vi "G4BaseTemplate_Singleton_4x4x4_GetInstance.vi"(8 "error in (no error)":errorcluster, 11 "reference in":refnum<class "G4BaseTemplate_Singleton_4x4x4.lvclass"> caption="This control should only be used when\na sub class is inheriting this class") -> (0 "error out":errorcluster, 1 "DVRRefOut":refnum<data-value>, 2 "NewObjectCreated":bool, 3 "reference out":refnum<class "G4BaseTemplate_Singleton_4x4x4.lvclass">, 5 "ObjectQueueName":string caption="This queue name could be used to destroy\nthe named queue that is used to hold the\nreference in the clean up.")   [LabVIEW 2014, in "G4BaseTemplate_Singleton_4x4x4.lvclass"]
uses:
  <resource>/Framework/Providers/Open_GDS/ClassProviders/Provider_EndevoGOOP400/Templates/G4BaseTemplate_Singleton_4x4x4/G4BaseTemplate_Singleton_4x4x4.lvclass
  <resource>/Framework/Providers/Open_GDS/ClassProviders/Provider_EndevoGOOP400/Templates/G4BaseTemplate_Singleton_4x4x4/protected/ObjectAttributes.ctl
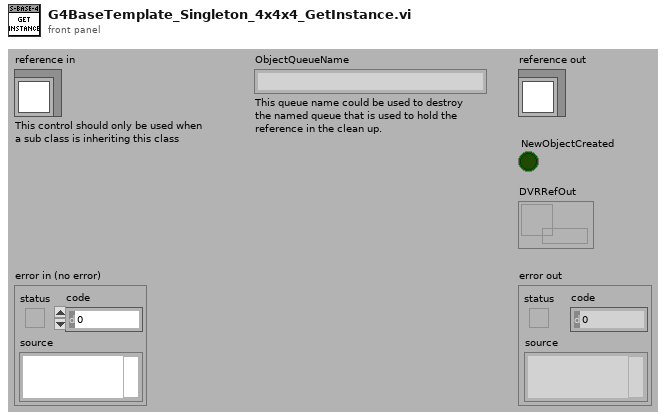
[diagram p1: front panel]
types:
  T1 = enum16{"Create or look up existing", "Look up existing"}
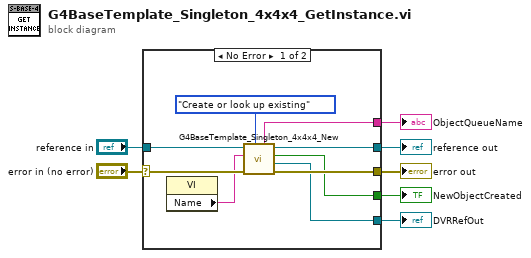
[diagram p0: block diagram]
diagram:
  n1 = case shown="No Error" "error in (no error)" {
    selector: "error in (no error)" -> [w15 w18]
    tunnel: [w16 w17] -> w7
    tunnel: [w14 w18] -> w5
    tunnel: "reference in" -> [w12 w17]
    tunnel: [w11 _] -> w3
    tunnel: [w10 _] -> w2
    tunnel: [w8 _] -> w1
    frame No Error {
      n2 = property class="VI"() -> ("Name"=w13:string)  [unwired: 2 in, 2 out]
      n3 = call <resource>:"G4BaseTemplate_Singleton_4x4x4_New.vi"("CreateMethod(Create or look up existing)"=T1."Create or look up existing", "error in (no error)"=w15, "Object name"=w13, "reference in"=w12) -> ("error out"=w14:errorcluster, "DVRRefOut"=w10:refnum<data-value>, "NewObjectCreated"=w11:bool, "reference out"=w16:refnum<class "G4BaseTemplate_Singleton_4x4x4.lvclass">, "ObjectQueueName"=w8:string)  [unwired: 3 in]
    }
    frame Error {
    }
  }
  "reference out" <- w7
  "error out" <- w5
  "NewObjectCreated" <- w3
  "DVRRefOut" <- w2
  "ObjectQueueName" <- w1
